vi "dvp Vi Set Noise Reduct3d State.vi"(10 "NoiseReduct3dState":i32, 11 "handle":u32) -> (3 "function return":u32(ring))   [LabVIEW 2018, in "LabViewDVPCamera.lvlib"]
doc: "LabviewDvp2Api dvpStatus dvpViSetNoiseReduct3dState(dvpHandle handle, BOOL NoiseReduct3dState);"
uses:
  LabViewDVPCamera.lvlib
  LabViewDVPCamera/LabViewDVPCamera.dll
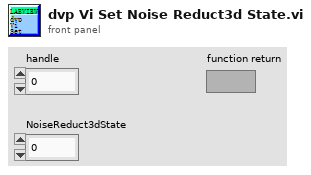
[diagram p1: front panel]
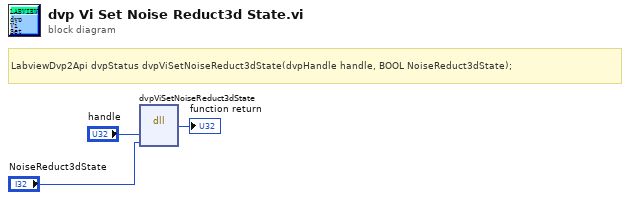
[diagram p0: block diagram]
diagram:
  # "LabviewDvp2Api dvpStatus dvpViSetNoiseReduct3dState(dvpHandle handle, BOOL NoiseReduct3dState);"
  n1 = dll-call lib="C:/Program Files (x86)/DVP2 Labview cn 64/Sample/LabViewDVPCamera/LabViewDVPCamera.*" fn="dvpViSetNoiseReduct3dState"("handle"="handle", "NoiseReduct3dState"="NoiseReduct3dState") -> (→"function return":u32)  [unwired: 5 in, 2 out]
